vi "OutputSwerveDrive.vi"() -> ()   [LabVIEW 2019]
doc: "This VI runs feedback and feedforward controllers, manages safety interlocks, and sends commands to the swerve drive motors. This VI also controls the commanded driver shifter (low gear or high gear) state."
uses:
  <vilib>/Rock Robotics/WPI/ThirdParty/Phoenix-LabVIEW/Motor Controller/Controls/CTRE_Phoenix_MotorControl_SupplyCurrentLimitConfiguration.ctl
  <vilib>/Rock Robotics/WPI/ThirdParty/Phoenix-LabVIEW/Motor Controller/Controls/CTRE_Phoenix_MotorControl_ControlMode.ctl
  <vilib>/Rock Robotics/WPI/Solenoid/WPI_SolenoidValue.ctl
  5bc46b9e-4d4b-4873-ab3e-533fd441fb60.vi
  eec0778c-44f4-445b-8f09-fbe21d33a92f.vi
  9255c0bb-7061-46f3-9b12-3c6a122af16e.vi
  4c0f1fb3-de9e-41af-b613-55c778746a69.vi
  1feddb54-1091-429e-8d95-9769f01e3028.vi
  9914bed3-0d1c-4b06-b050-22aab9a27a8c.vi
  outputs.vi
  dsdata.vi
  sensors.vi
  refnums.vi
  GRNF_CTREMotor.vi
  <vilib>/Rock Robotics/WPI/ThirdParty/Phoenix-LabVIEW/Motor Controller/Get/CTRE_Phoenix_MotorController_GetSelectedSensorData.vi
  robotprofile.vi
  TAI_Motor.vi
  GRNF_GenericSolenoid.vi
  TAI_Solenoid.vi
  <vilib>/Rock Robotics/WPI/Solenoid/WPI_SolenoidSetEnum.vi
panel:
  in  "Decceleration Limit (/s)":dbl=50.0
  in  "Acceleration Limit (/s)":dbl=2.0
  in  "Force to Low Gear":bool
  in  "Force To High Gear":bool
  in  "Drive Command Override [0,1]":dbl
  in  "Manually Override Drive Calibration":bool
  in  "Time Below Speed (ms)":u32=100
  in  "Time Above Speed (ms)":u32=100
  in  "Switch to Low Gear (rpm)":dbl=740.0
  in  "Switch to High Gear (rpm)":dbl=2000.0
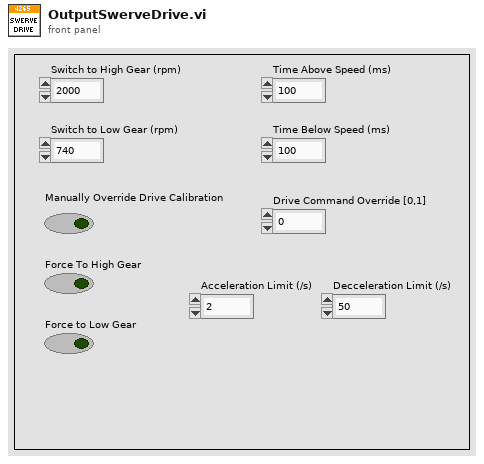
[diagram p1: front panel]
types:
  T1 = enum16{"Driver Control", "Auto Targeting", "Feeder Station"}
  T2 = typedef "CTRE_Phoenix_MotorControl_ControlMode.ctl" = u16
  T3 = typedef "CTRE_Phoenix_MotorControl_SupplyCurrentLimitConfiguration.ctl" = cluster{"Enable?":bool, "Current Limit":dbl, "Threshold Current":dbl, "Threshold Time":dbl}
  T4 = typedef "WPI_MotorControlDeviceRef.ctl" = cluster{"DeviceStatus":errorcluster, "Type":T5, "PWM":cluster{"PWM Channel":T6, "DeadBand":T7}, "CAN":cluster{"Device Number":u8, "SetOutput VI Ref":variant, "GetOutput VI Ref":variant, "Enable VI Ref":variant, "Disable VI Ref":variant, "Data":variant}, "Invert":bool, "DIO PWM":cluster{"PWM \"Enable\" Channel":T6, "DIOChannel":T8, "PWM Rate":dbl}}
  T5 = typedef "WPI_MotorControlType.ctl" = enum16{"PWM", "CAN", "DIO PWM"}
  T6 = typedef "FPGA_DIOPWMChannel.ctl" = enum8{"PWM 0", "PWM 1", "PWM 2", "PWM 3", "PWM 4", "PWM 5", "PWM 6", "PWM 7", "PWM 8", "PWM 9", "PWM MXP 0", "PWM MXP 1", "PWM MXP 2", "PWM MXP 3", "PWM MXP 4", "PWM MXP 5", "PWM MXP 6", "PWM MXP 7", "PWM MXP 8", "PWM MXP 9", "Invalid"}
  T7 = typedef "WPI_PWMDeadband.ctl" = cluster{"Name":string, "maxPositivePwm":i32, "minPositivePwm":i32, "centerPwm":i32, "maxNegativePwm":i32, "minNegativePwm":i32, "angularRange":u16}
  T8 = typedef "FPGA_DIOChannel.ctl" = enum8{"DIO 0", "DIO 1", "DIO 2", "DIO 3", "DIO 4", "DIO 5", "DIO 6", "DIO 7", "DIO 8", "DIO 9", "DIO MXP 0", "DIO MXP 1", "DIO MXP 2", "DIO MXP 3", "DIO MXP 4", "DIO MXP 5", "DIO MXP 6", "DIO MXP 7", "DIO MXP 8", "DIO MXP 9", "DIO MXP 10", "DIO MXP 11", "DIO MXP 12", "DIO MXP 13", "DIO MXP 14", "DIO MXP 15", "SPI Port CS1", "SPI Port CS2", "SPI Port CS3", "SPI Port MISO", "SPI Port MOSI", "Invalid"}
  T9 = enum16{"Low Gear", "High Gear", "Transiting", "Unknown", "Force Low Gear"}
  T10 = typedef "WPI_SolenoidDevRef.ctl" = cluster{"DevStatus":errorcluster, "Pneumatics Control Module":u8, "Forward Solenoid Channel":T11, "Reverse Solenoid Channel":T11}
  T11 = typedef "WPI_SolenoidChannel.ctl" = enum8{"Solenoid 0", "Solenoid 1", "Solenoid 2", "Solenoid 3", "Solenoid 4", "Solenoid 5", "Solenoid 6", "Solenoid 7", "Invalid"}
  T12 = typedef "WPI_SolenoidValue.ctl" = enum16{"Off", "On", "Forward", "Reverse"}
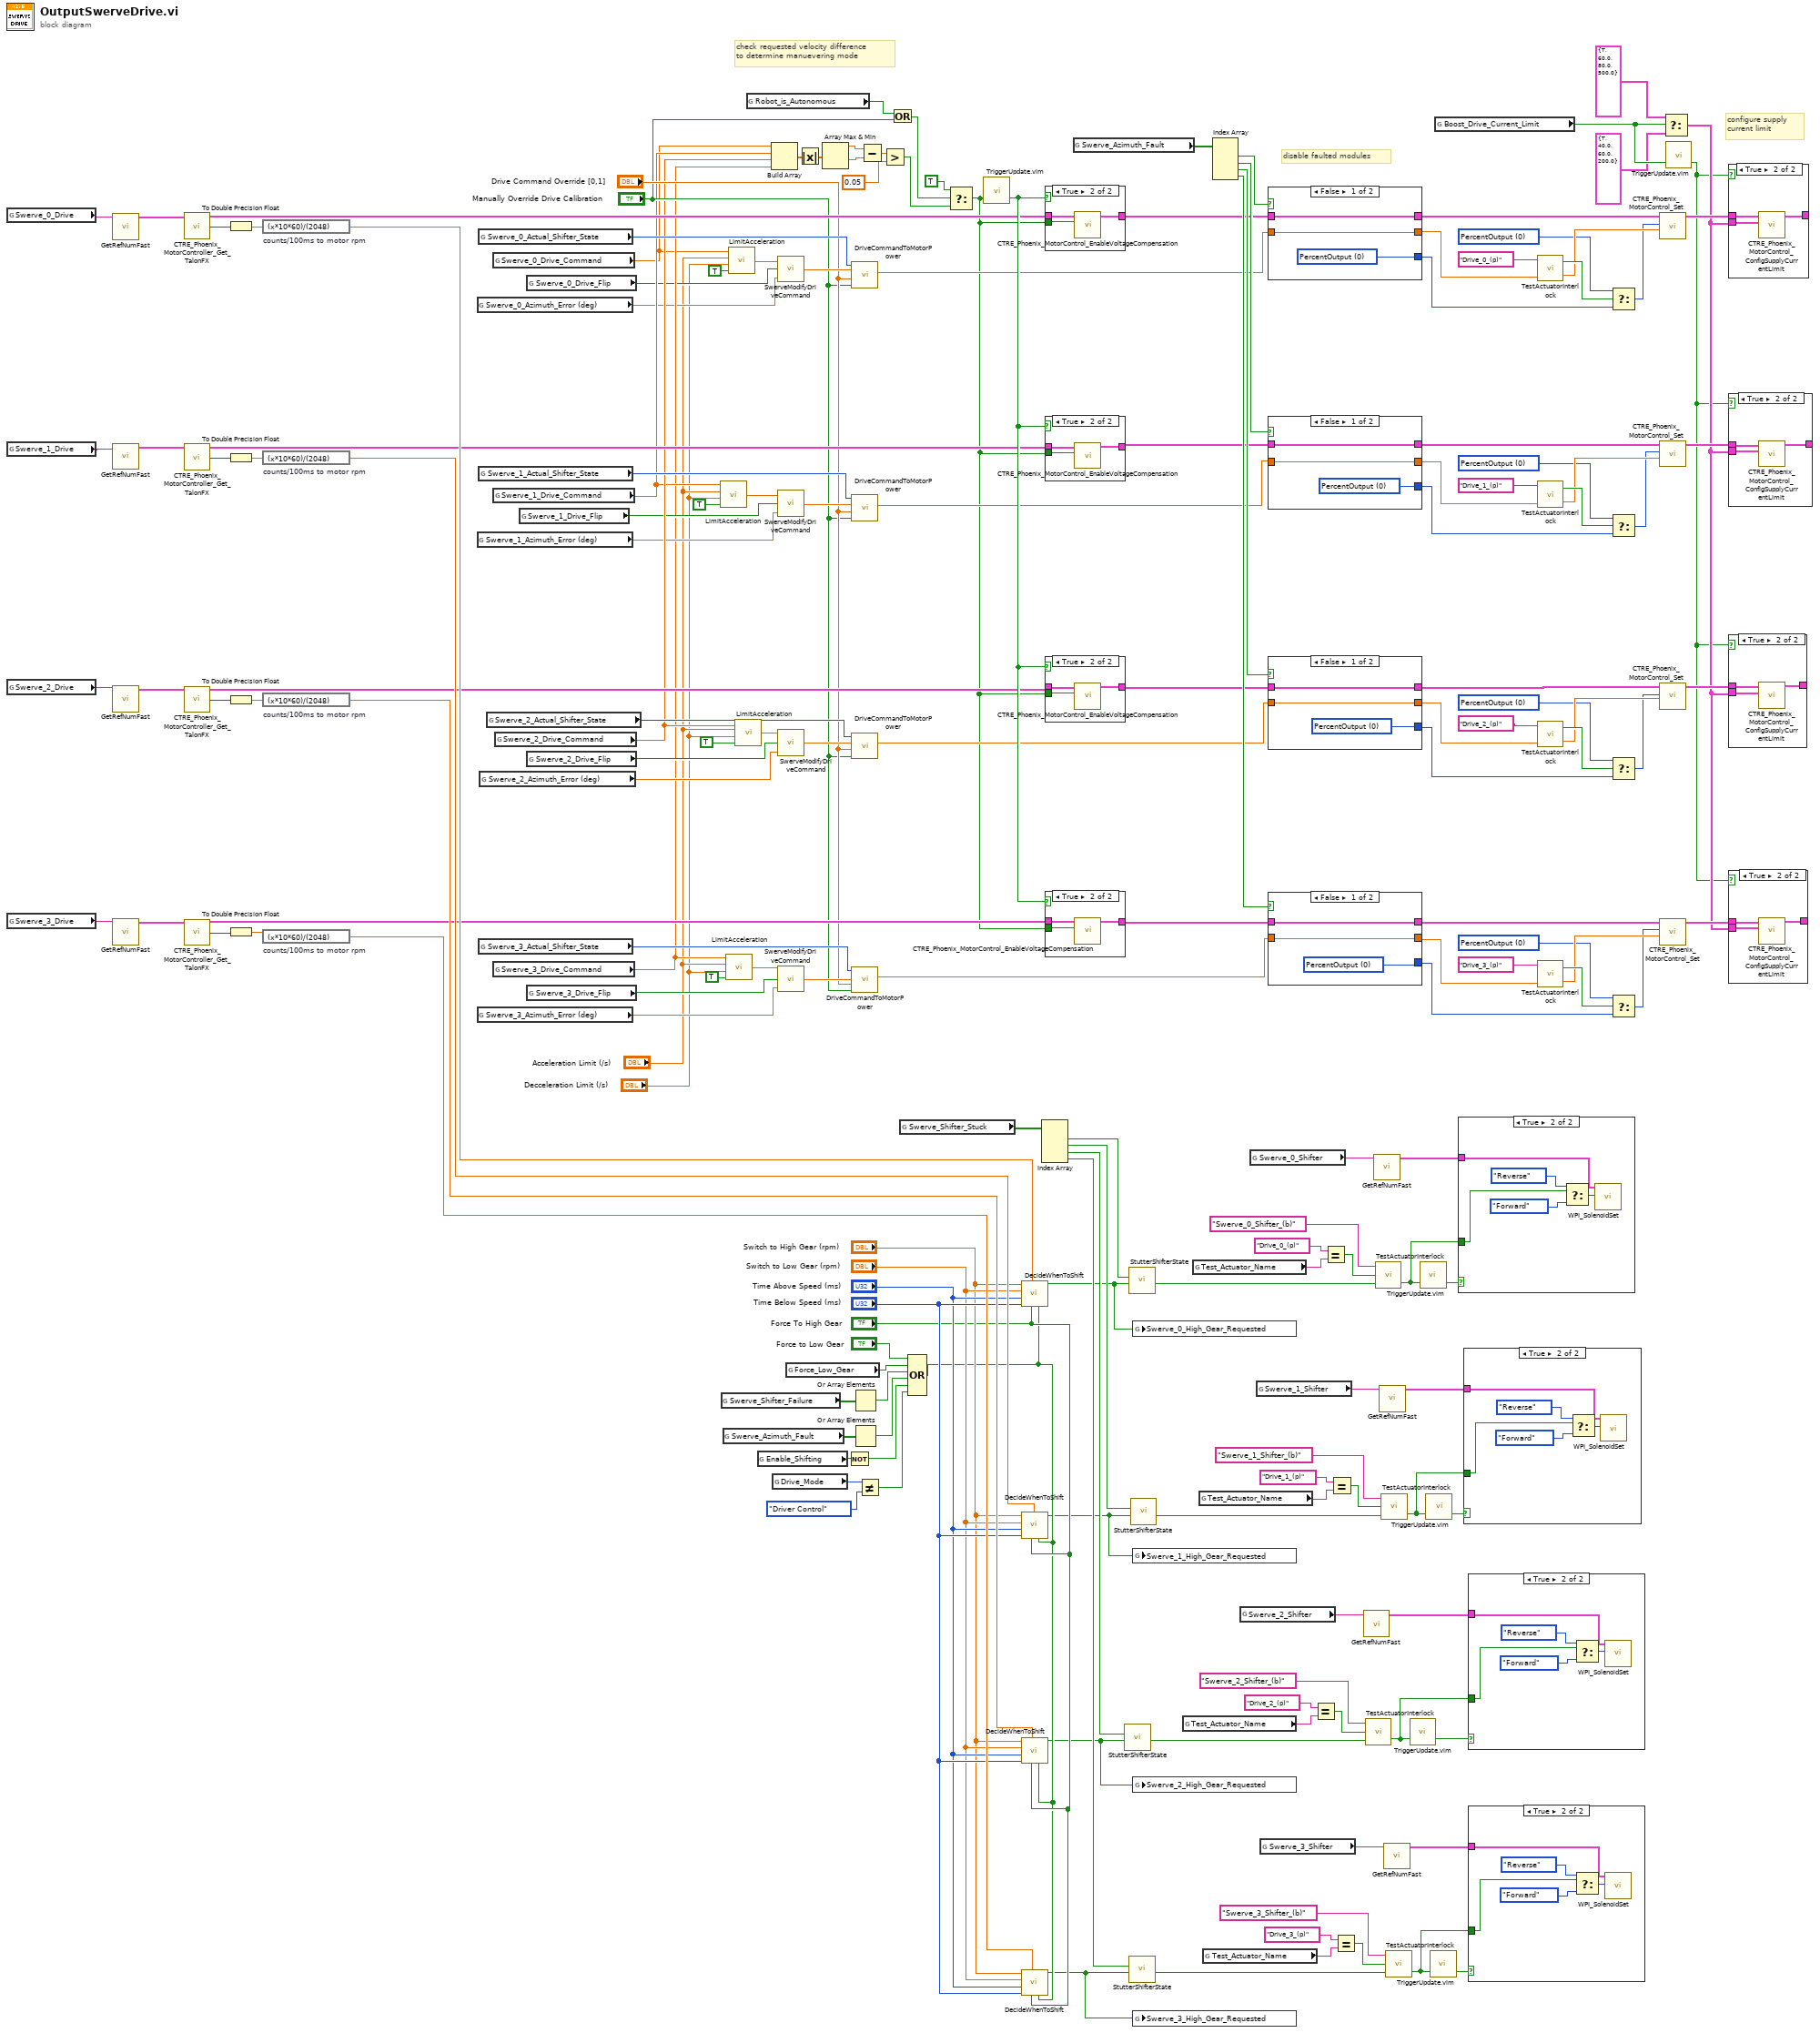
[diagram p0: block diagram]
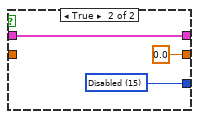
[diagram p14: hidden frame]
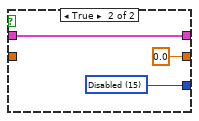
[diagram p15: hidden frame]
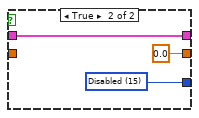
[diagram p16: hidden frame]
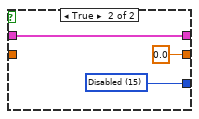
[diagram p17: hidden frame]
diagram:
  w146 = T2 0 items=["PercentOutput"=0, "Position"=1, "Velocity"=2, "Current"=3, "Follower"=5, "MotionProfile"=6, "MotionMagic"=7, "MotionProfileArc"=10, "Disabled"=15] ("Control Mode")
  w155 = T2 0 items=["PercentOutput"=0, "Position"=1, "Velocity"=2, "Current"=3, "Follower"=5, "MotionProfile"=6, "MotionMagic"=7, "MotionProfileArc"=10, "Disabled"=15] ("Control Mode")
  w164 = T2 0 items=["PercentOutput"=0, "Position"=1, "Velocity"=2, "Current"=3, "Follower"=5, "MotionProfile"=6, "MotionMagic"=7, "MotionProfileArc"=10, "Disabled"=15] ("Control Mode")
  w173 = T2 0 items=["PercentOutput"=0, "Position"=1, "Velocity"=2, "Current"=3, "Follower"=5, "MotionProfile"=6, "MotionMagic"=7, "MotionProfileArc"=10, "Disabled"=15] ("Control Mode")
  # "check requested velocity difference\nto determine manuevering mode"
  # "configure supply\ncurrent limit"
  # "disable faulted modules"
  n1 = global read "refnums.vi" "Swerve_0_Drive"() -> (w152:string)
  n2 = global read "refnums.vi" "Swerve_1_Drive"() -> (w161:string)
  n3 = global read "refnums.vi" "Swerve_2_Drive"() -> (w170:string)
  n4 = global read "refnums.vi" "Swerve_3_Drive"() -> (w179:string)
  n5 = call-poly "GetRefNumFast.vi"("RefNum Name"=w152) -> ("Device Reference"=w111:T4)  [unwired: 5 in, 1 out]
  n6 = call-poly "GetRefNumFast.vi"("RefNum Name"=w161) -> ("Device Reference"=w110:T4)  [unwired: 5 in, 1 out]
  n7 = call-poly "GetRefNumFast.vi"("RefNum Name"=w170) -> ("Device Reference"=w109:T4)  [unwired: 5 in, 1 out]
  n8 = call-poly "GetRefNumFast.vi"("RefNum Name"=w179) -> ("Device Reference"=w108:T4)  [unwired: 5 in, 1 out]
  n9 = call-poly <vilib>:"CTRE_Phoenix_MotorController_Get_TalonFX.vi"("PhoenixMotorControlDevRef"=w111) -> ("PhoenixMotorControlDevRef"=w114:T4, "Velocity (Raw Sensor Units per 100 ms)"=w119:i32)  [unwired: 11 in, 2 out]
  n10 = call-poly <vilib>:"CTRE_Phoenix_MotorController_Get_TalonFX.vi"("PhoenixMotorControlDevRef"=w110) -> ("PhoenixMotorControlDevRef"=w112:T4, "Velocity (Raw Sensor Units per 100 ms)"=w118:i32)  [unwired: 11 in, 2 out]
  n11 = call-poly <vilib>:"CTRE_Phoenix_MotorController_Get_TalonFX.vi"("PhoenixMotorControlDevRef"=w109) -> ("PhoenixMotorControlDevRef"=w113:T4, "Velocity (Raw Sensor Units per 100 ms)"=w117:i32)  [unwired: 11 in, 2 out]
  n12 = call-poly <vilib>:"CTRE_Phoenix_MotorController_Get_TalonFX.vi"("PhoenixMotorControlDevRef"=w108) -> ("PhoenixMotorControlDevRef"=w103:T4, "Velocity (Raw Sensor Units per 100 ms)"=w116:i32)  [unwired: 11 in, 2 out]
  n13 = To Double Precision Float(number=w119) -> (double precision float=w126:dbl)
  n14 = To Double Precision Float(number=w118) -> (double precision float=w125:dbl)
  n15 = To Double Precision Float(number=w117) -> (double precision float=w124:dbl)
  n16 = To Double Precision Float(number=w116) -> (double precision float=w123:dbl)
  n17 = expression code="(x*10*60)/(2048)" "counts/100ms to motor rpm"(w126) -> (w120:dbl)
  n18 = expression code="(x*10*60)/(2048)" "counts/100ms to motor rpm"(w125) -> (w121:dbl)
  n19 = expression code="(x*10*60)/(2048)" "counts/100ms to motor rpm"(w124) -> (w122:dbl)
  n20 = expression code="(x*10*60)/(2048)" "counts/100ms to motor rpm"(w123) -> (w134:dbl)
  n21 = global read "outputs.vi" "Swerve_0_Azimuth_Error (deg)"() -> (w70:dbl)
  n22 = global read "outputs.vi" "Swerve_1_Azimuth_Error (deg)"() -> (w76:dbl)
  n23 = global read "outputs.vi" "Swerve_3_Azimuth_Error (deg)"() -> (w115:dbl)
  n24 = global read "sensors.vi" "Swerve_0_Actual_Shifter_State"() -> (w99:T9)
  n25 = global read "sensors.vi" "Swerve_1_Actual_Shifter_State"() -> (w96:T9)
  n26 = global read "sensors.vi" "Swerve_3_Actual_Shifter_State"() -> (w90:T9)
  n27 = global read "outputs.vi" "Swerve_2_Azimuth_Error (deg)"() -> (w81:dbl)
  n28 = global read "sensors.vi" "Swerve_2_Actual_Shifter_State"() -> (w94:T9)
  n29 = global read "outputs.vi" "Swerve_0_Drive_Command"() -> (w67:dbl)
  n30 = global read "outputs.vi" "Swerve_1_Drive_Command"() -> (w75:dbl)
  n31 = global read "outputs.vi" "Swerve_3_Drive_Command"() -> (w72:dbl)
  n32 = global read "outputs.vi" "Swerve_2_Drive_Command"() -> (w84:dbl)
  n33 = global read "outputs.vi" "Swerve_1_Drive_Flip"() -> (w78:bool)
  n34 = global read "outputs.vi" "Swerve_0_Drive_Flip"() -> (w69:bool)
  n35 = global read "outputs.vi" "Swerve_2_Drive_Flip"() -> (w79:bool)
  n36 = global read "outputs.vi" "Swerve_3_Drive_Flip"() -> (w74:bool)
  n37 = call "LimitAcceleration.vi"("Apply Limit"=TRUE, "Decceleration Limit (/s)"="Decceleration Limit (/s)", "Acceleration Limit (/s)"="Acceleration Limit (/s)", "Raw Input"=w75) -> ("Output"=w77:dbl)
  n38 = global read "sensors.vi" "Swerve_Shifter_Failure"() -> (w23:bool[])
  n39 = global read "sensors.vi" "Swerve_Azimuth_Fault"() -> (w21:bool[])
  n40 = call "LimitAcceleration.vi"("Apply Limit"=TRUE, "Decceleration Limit (/s)"="Decceleration Limit (/s)", "Acceleration Limit (/s)"="Acceleration Limit (/s)", "Raw Input"=w72) -> ("Output"=w73:dbl)
  n41 = call "LimitAcceleration.vi"("Apply Limit"=TRUE, "Decceleration Limit (/s)"="Decceleration Limit (/s)", "Acceleration Limit (/s)"="Acceleration Limit (/s)", "Raw Input"=w67) -> ("Output"=w68:dbl)
  n42 = call "LimitAcceleration.vi"("Apply Limit"=TRUE, "Decceleration Limit (/s)"="Decceleration Limit (/s)", "Acceleration Limit (/s)"="Acceleration Limit (/s)", "Raw Input"=w84) -> ("Output"=w82:dbl)
  n43 = global read "dsdata.vi" "Robot_is_Autonomous"() -> (w86:bool)
  n44 = global read "robotprofile.vi" "Enable_Shifting"() -> (w10:bool)
  n45 = Build Array(w67, w75, w84, w72) -> (w133:dbl[])
  n46 = global read "outputs.vi" "Drive_Mode"() -> (w3:T1)
  n47 = call "SwerveModifyDriveCommand.vi"("Azimuth Error (deg)"=w70, "Flip Drive Command"=w69, "Raw Drive Command (ul)"=w68) -> ("Modified Drive Command (ul)"=w100:dbl)
  n48 = call "SwerveModifyDriveCommand.vi"("Azimuth Error (deg)"=w76, "Flip Drive Command"=w78, "Raw Drive Command (ul)"=w77) -> ("Modified Drive Command (ul)"=w97:dbl)
  n49 = call "SwerveModifyDriveCommand.vi"("Azimuth Error (deg)"=w81, "Flip Drive Command"=w79, "Raw Drive Command (ul)"=w82) -> ("Modified Drive Command (ul)"=w93:dbl)
  n50 = call "SwerveModifyDriveCommand.vi"("Azimuth Error (deg)"=w115, "Flip Drive Command"=w74, "Raw Drive Command (ul)"=w73) -> ("Modified Drive Command (ul)"=w91:dbl)
  n51 = global read "outputs.vi" "Force_Low_Gear"() -> (w24:bool)
  n52 = Absolute Value(x=w133) -> (abs(x)=w127:dbl[])
  n53 = Array Max & Min(array=w127) -> (max value=w132:dbl, min value=w131:dbl)  [unwired: 2 out]
  n54 = Not(x=w10) -> (.not. x?=w9:bool)
  n55 = call "DriveCommandToMotorPower.vi"("Drive Command Override"="Manually Override Drive Calibration", "Drive Command Override (ul) [-1,1]"="Drive Command Override [0,1]", "Drive Command (ul) [-1,1]"=w100, "Actual Shifter State"=w99) -> ("Motor Power (ul) [-1,1]"=w98:dbl)  [unwired: 7 in]
  n56 = call "DriveCommandToMotorPower.vi"("Drive Command Override"="Manually Override Drive Calibration", "Drive Command Override (ul) [-1,1]"="Drive Command Override [0,1]", "Drive Command (ul) [-1,1]"=w97, "Actual Shifter State"=w96) -> ("Motor Power (ul) [-1,1]"=w95:dbl)  [unwired: 7 in]
  n57 = call "DriveCommandToMotorPower.vi"("Drive Command Override"="Manually Override Drive Calibration", "Drive Command Override (ul) [-1,1]"="Drive Command Override [0,1]", "Drive Command (ul) [-1,1]"=w93, "Actual Shifter State"=w94) -> ("Motor Power (ul) [-1,1]"=w92:dbl)  [unwired: 7 in]
  n58 = call "DriveCommandToMotorPower.vi"("Drive Command Override"="Manually Override Drive Calibration", "Drive Command Override (ul) [-1,1]"="Drive Command Override [0,1]", "Drive Command (ul) [-1,1]"=w91, "Actual Shifter State"=w90) -> ("Motor Power (ul) [-1,1]"=w89:dbl)  [unwired: 7 in]
  n59 = Or Array Elements(Boolean array=w23) -> (logical OR=w22:bool)
  n60 = Or Array Elements(Boolean array=w21) -> (logical OR=w20:bool)
  n61 = Not Equal?(x=w3, y=T1."Driver Control") -> (x != y?=w1:bool)
  n62 = Subtract(x=w132, y=w131) -> (x-y=w130:dbl)
  n63 = Greater?(x=w130, y=0.05) -> (0:w101:bool)
  n64 = Or(x=w86, y="Manually Override Drive Calibration") -> (x .or. y?=w87:bool)
  n65 = global read "sensors.vi" "Swerve_Shifter_Stuck"() -> (w18:bool[])
  n66 = Compound Arithmetic op=OR("Force to Low Gear", w24, w22, w20, w9, w1) -> (w25:bool)
  n67 = Select(t=TRUE, s=w87, f=w101) -> (s? t:f=w4:bool)
  n68 = call "TriggerUpdate.vim"("Trigger"=w4) -> ("Update"=w128:bool)  [unwired: 2 in]
  n69 = call "DecideWhenToShift.vi"("Force to Low Gear"=w25, "Force To High Gear"="Force To High Gear", "Drive Motor Speed (rpm)"=w120, "Time Below Speed (ms)"="Time Below Speed (ms)", "Time Above Speed (ms)"="Time Above Speed (ms)", "Switch to Low Gear (rpm)"="Switch to Low Gear (rpm)", "Switch to High Gear (rpm)"="Switch to High Gear (rpm)") -> ("Requested Shifter State"=w7:bool)  [unwired: 4 in]
  n70 = call "DecideWhenToShift.vi"("Force to Low Gear"=w25, "Force To High Gear"="Force To High Gear", "Drive Motor Speed (rpm)"=w121, "Time Below Speed (ms)"="Time Below Speed (ms)", "Time Above Speed (ms)"="Time Above Speed (ms)", "Switch to Low Gear (rpm)"="Switch to Low Gear (rpm)", "Switch to High Gear (rpm)"="Switch to High Gear (rpm)") -> ("Requested Shifter State"=w8:bool)  [unwired: 4 in]
  n71 = call "DecideWhenToShift.vi"("Force to Low Gear"=w25, "Force To High Gear"="Force To High Gear", "Drive Motor Speed (rpm)"=w122, "Time Below Speed (ms)"="Time Below Speed (ms)", "Time Above Speed (ms)"="Time Above Speed (ms)", "Switch to Low Gear (rpm)"="Switch to Low Gear (rpm)", "Switch to High Gear (rpm)"="Switch to High Gear (rpm)") -> ("Requested Shifter State"=w6:bool)  [unwired: 4 in]
  n72 = call "DecideWhenToShift.vi"("Force to Low Gear"=w25, "Force To High Gear"="Force To High Gear", "Drive Motor Speed (rpm)"=w134, "Time Below Speed (ms)"="Time Below Speed (ms)", "Time Above Speed (ms)"="Time Above Speed (ms)", "Switch to Low Gear (rpm)"="Switch to Low Gear (rpm)", "Switch to High Gear (rpm)"="Switch to High Gear (rpm)") -> ("Requested Shifter State"=w5:bool)  [unwired: 4 in]
  n73 = Index Array(array=w18) -> (element #1=w16:bool, element #2=w14:bool, element #3=w13:bool, element #4=w11:bool)  [unwired: 4 in]
  n74 = case shown="True" w128 {
    tunnel: w114 -> [w185 w188]
    tunnel: [w185 w187] -> w107
    tunnel: w4 -> [_ w186]
    frame False {
    }
    frame True {
      n75 = call <vilib>:"CTRE_Phoenix_MotorControl_EnableVoltageCompensation.vi"("Enable Voltage Compensation?"=w186, "PhoenixMotorControlDevRef"=w188) -> ("PhoenixMotorControlDevRef"=w187:T4)  [unwired: 8 in, 1 out]
    }
  }
  n76 = case shown="True" w128 {
    tunnel: w112 -> [w189 w192]
    tunnel: [w189 w191] -> w106
    tunnel: w4 -> [_ w190]
    frame False {
    }
    frame True {
      n77 = call <vilib>:"CTRE_Phoenix_MotorControl_EnableVoltageCompensation.vi"("Enable Voltage Compensation?"=w190, "PhoenixMotorControlDevRef"=w192) -> ("PhoenixMotorControlDevRef"=w191:T4)  [unwired: 8 in, 1 out]
    }
  }
  n78 = case shown="True" w128 {
    tunnel: w113 -> [w193 w196]
    tunnel: [w193 w195] -> w105
    tunnel: w4 -> [_ w194]
    frame False {
    }
    frame True {
      n79 = call <vilib>:"CTRE_Phoenix_MotorControl_EnableVoltageCompensation.vi"("Enable Voltage Compensation?"=w194, "PhoenixMotorControlDevRef"=w196) -> ("PhoenixMotorControlDevRef"=w195:T4)  [unwired: 8 in, 1 out]
    }
  }
  n80 = case shown="True" w128 {
    tunnel: [w197 w200] -> w104
    tunnel: w4 -> [_ w199]
    tunnel: w103 -> [w197 w198]
    frame False {
    }
    frame True {
      n81 = call <vilib>:"CTRE_Phoenix_MotorControl_EnableVoltageCompensation.vi"("Enable Voltage Compensation?"=w199, "PhoenixMotorControlDevRef"=w198) -> ("PhoenixMotorControlDevRef"=w200:T4)  [unwired: 8 in, 1 out]
    }
  }
  n82 = global read "sensors.vi" "Swerve_Azimuth_Fault"() -> (w184:bool[])
  n83 = call "StutterShifterState.vi"("Requested Shifter State"=w6, "Request Stutter"=w13) -> ("Stuttered Shifter State"=w19:bool)  [unwired: 9 in]
  n84 = call "StutterShifterState.vi"("Requested Shifter State"=w7, "Request Stutter"=w16) -> ("Stuttered Shifter State"=w17:bool)  [unwired: 9 in]
  n85 = call "StutterShifterState.vi"("Requested Shifter State"=w5, "Request Stutter"=w11) -> ("Stuttered Shifter State"=w12:bool)  [unwired: 9 in]
  n86 = call "StutterShifterState.vi"("Requested Shifter State"=w8, "Request Stutter"=w14) -> ("Stuttered Shifter State"=w15:bool)  [unwired: 9 in]
  n87 = global write "outputs.vi" "Swerve_0_High_Gear_Requested"(w7) -> ()
  n88 = global write "outputs.vi" "Swerve_1_High_Gear_Requested"(w8) -> ()
  n89 = global write "outputs.vi" "Swerve_2_High_Gear_Requested"(w6) -> ()
  n90 = global write "outputs.vi" "Swerve_3_High_Gear_Requested"(w5) -> ()
  n91 = global read "dsdata.vi" "Test_Actuator_Name"() -> (w41:string)
  n92 = global read "dsdata.vi" "Test_Actuator_Name"() -> (w57:string)
  n93 = global read "dsdata.vi" "Test_Actuator_Name"() -> (w49:string)
  n94 = global read "dsdata.vi" "Test_Actuator_Name"() -> (w33:string)
  n95 = Index Array(array=w184) -> (element #1=w143:bool, element #2=w142:bool, element #3=w141:bool, element #4=w183:bool)  [unwired: 4 in]
  n96 = global read "refnums.vi" "Swerve_2_Shifter"() -> (w43:string)
  n97 = global read "refnums.vi" "Swerve_0_Shifter"() -> (w59:string)
  n98 = global read "refnums.vi" "Swerve_1_Shifter"() -> (w51:string)
  n99 = global read "refnums.vi" "Swerve_3_Shifter"() -> (w35:string)
  n100 = case shown="False" w143 {
    tunnel: [w203 w206] -> w151
    tunnel: w107 -> [w203 w206]
    tunnel: [w202 0.0 ("Command")] -> w148
    tunnel: w98 -> [w202 _]
    tunnel: [w201 w204] -> w145
    frame False {
      w201 = T2 0 items=["PercentOutput"=0, "Position"=1, "Velocity"=2, "Current"=3, "Follower"=5, "MotionProfile"=6, "MotionMagic"=7, "MotionProfileArc"=10, "Disabled"=15] ("Control Mode")
    }
    frame True {
      w204 = T2 15 items=["PercentOutput"=0, "Position"=1, "Velocity"=2, "Current"=3, "Follower"=5, "MotionProfile"=6, "MotionMagic"=7, "MotionProfileArc"=10, "Disabled"=15] ("Control Mode")
    }
  }
  n101 = case shown="False" w142 {
    tunnel: [w209 w212] -> w160
    tunnel: w106 -> [w209 w212]
    tunnel: [w208 0.0 ("Command")] -> w157
    tunnel: w95 -> [w208 _]
    tunnel: [w207 w210] -> w154
    frame False {
      w207 = T2 0 items=["PercentOutput"=0, "Position"=1, "Velocity"=2, "Current"=3, "Follower"=5, "MotionProfile"=6, "MotionMagic"=7, "MotionProfileArc"=10, "Disabled"=15] ("Control Mode")
    }
    frame True {
      w210 = T2 15 items=["PercentOutput"=0, "Position"=1, "Velocity"=2, "Current"=3, "Follower"=5, "MotionProfile"=6, "MotionMagic"=7, "MotionProfileArc"=10, "Disabled"=15] ("Control Mode")
    }
  }
  n102 = case shown="False" w141 {
    tunnel: [w215 w218] -> w169
    tunnel: w105 -> [w215 w218]
    tunnel: [w214 0.0 ("Command")] -> w166
    tunnel: w92 -> [w214 _]
    tunnel: [w213 w216] -> w163
    frame False {
      w213 = T2 0 items=["PercentOutput"=0, "Position"=1, "Velocity"=2, "Current"=3, "Follower"=5, "MotionProfile"=6, "MotionMagic"=7, "MotionProfileArc"=10, "Disabled"=15] ("Control Mode")
    }
    frame True {
      w216 = T2 15 items=["PercentOutput"=0, "Position"=1, "Velocity"=2, "Current"=3, "Follower"=5, "MotionProfile"=6, "MotionMagic"=7, "MotionProfileArc"=10, "Disabled"=15] ("Control Mode")
    }
  }
  n103 = case shown="False" w183 {
    tunnel: [w221 w224] -> w178
    tunnel: w104 -> [w221 w224]
    tunnel: [w220 0.0 ("Command")] -> w175
    tunnel: w89 -> [w220 _]
    tunnel: [w219 w222] -> w172
    frame False {
      w219 = T2 0 items=["PercentOutput"=0, "Position"=1, "Velocity"=2, "Current"=3, "Follower"=5, "MotionProfile"=6, "MotionMagic"=7, "MotionProfileArc"=10, "Disabled"=15] ("Control Mode")
    }
    frame True {
      w222 = T2 15 items=["PercentOutput"=0, "Position"=1, "Velocity"=2, "Current"=3, "Follower"=5, "MotionProfile"=6, "MotionMagic"=7, "MotionProfileArc"=10, "Disabled"=15] ("Control Mode")
    }
  }
  n104 = Equal?(x="Drive_2_(p)" ("Actuator_Name"), y=w41) -> (x = y?=w40:bool)
  n105 = Equal?(x="Drive_0_(p)" ("Actuator_Name"), y=w57) -> (x = y?=w56:bool)
  n106 = Equal?(x="Drive_1_(p)" ("Actuator_Name"), y=w49) -> (x = y?=w48:bool)
  n107 = Equal?(x="Drive_3_(p)" ("Actuator_Name"), y=w33) -> (x = y?=w32:bool)
  n108 = call-poly "GetRefNumFast.vi"("RefNum Name"=w43) -> ("Device Reference"=w45:T10)  [unwired: 5 in, 1 out]
  n109 = call-poly "TestActuatorInterlock.vi"("Normal Output"=w19, "Override Actuator Bypass"=w40, "Actuator Name"="Swerve_2_Shifter_(b)" ("Actuator_Name")) -> ("Interlock Output"=w46:bool)  [unwired: 1 out]
  n110 = call-poly "GetRefNumFast.vi"("RefNum Name"=w59) -> ("Device Reference"=w61:T10)  [unwired: 5 in, 1 out]
  n111 = call-poly "TestActuatorInterlock.vi"("Normal Output"=w17, "Override Actuator Bypass"=w56, "Actuator Name"="Swerve_0_Shifter_(b)" ("Actuator_Name")) -> ("Interlock Output"=w62:bool)  [unwired: 1 out]
  n112 = call-poly "GetRefNumFast.vi"("RefNum Name"=w51) -> ("Device Reference"=w53:T10)  [unwired: 5 in, 1 out]
  n113 = call-poly "TestActuatorInterlock.vi"("Normal Output"=w15, "Override Actuator Bypass"=w48, "Actuator Name"="Swerve_1_Shifter_(b)" ("Actuator_Name")) -> ("Interlock Output"=w54:bool)  [unwired: 1 out]
  n114 = call-poly "GetRefNumFast.vi"("RefNum Name"=w35) -> ("Device Reference"=w37:T10)  [unwired: 5 in, 1 out]
  n115 = call-poly "TestActuatorInterlock.vi"("Normal Output"=w12, "Override Actuator Bypass"=w32, "Actuator Name"="Swerve_3_Shifter_(b)" ("Actuator_Name")) -> ("Interlock Output"=w38:bool)  [unwired: 1 out]
  n116 = call "TriggerUpdate.vim"("Trigger"=w46) -> ("Update"=w47:bool)  [unwired: 2 in]
  n117 = call "TriggerUpdate.vim"("Trigger"=w62) -> ("Update"=w63:bool)  [unwired: 2 in]
  n118 = call "TriggerUpdate.vim"("Trigger"=w54) -> ("Update"=w55:bool)  [unwired: 2 in]
  n119 = call "TriggerUpdate.vim"("Trigger"=w38) -> ("Update"=w39:bool)  [unwired: 2 in]
  n120 = global read "outputs.vi" "Boost_Drive_Current_Limit"() -> (w181:bool)
  n121 = case shown="True" w63 {
    tunnel: w61 -> [_ w229]
    tunnel: w62 -> [_ w228]
    frame False {
    }
    frame True {
      n122 = Select(t=WPI_SolenoidValue."Reverse" ("Value"), s=w228, f=WPI_SolenoidValue."Forward" ("Value")) -> (s? t:f=w225:T12)
      n123 = call-poly <vilib>:"WPI_SolenoidSet.vi"("Value"=w225, "SolenoidDevRef"=w229) -> ()  [unwired: 8 in, 2 out]
    }
  }
  n124 = case shown="True" w55 {
    tunnel: w53 -> [_ w234]
    tunnel: w54 -> [_ w233]
    frame False {
    }
    frame True {
      n125 = Select(t=WPI_SolenoidValue."Reverse" ("Value"), s=w233, f=WPI_SolenoidValue."Forward" ("Value")) -> (s? t:f=w230:T12)
      n126 = call-poly <vilib>:"WPI_SolenoidSet.vi"("Value"=w230, "SolenoidDevRef"=w234) -> ()  [unwired: 8 in, 2 out]
    }
  }
  n127 = case shown="True" w47 {
    tunnel: w45 -> [_ w239]
    tunnel: w46 -> [_ w238]
    frame False {
    }
    frame True {
      n128 = Select(t=WPI_SolenoidValue."Reverse" ("Value"), s=w238, f=WPI_SolenoidValue."Forward" ("Value")) -> (s? t:f=w235:T12)
      n129 = call-poly <vilib>:"WPI_SolenoidSet.vi"("Value"=w235, "SolenoidDevRef"=w239) -> ()  [unwired: 8 in, 2 out]
    }
  }
  n130 = case shown="True" w39 {
    tunnel: w37 -> [_ w244]
    tunnel: w38 -> [_ w243]
    frame False {
    }
    frame True {
      n131 = Select(t=WPI_SolenoidValue."Reverse" ("Value"), s=w243, f=WPI_SolenoidValue."Forward" ("Value")) -> (s? t:f=w240:T12)
      n132 = call-poly <vilib>:"WPI_SolenoidSet.vi"("Value"=w240, "SolenoidDevRef"=w244) -> ()  [unwired: 8 in, 2 out]
    }
  }
  n133 = call-poly "TestActuatorInterlock.vi"("Normal Output"=w148, "Actuator Name"="Drive_0_(p)" ("Actuator_Name")) -> ("Interlock Output"=w147:dbl, "Testing This Actuator"=w150:bool)  [unwired: 1 in]
  n134 = call-poly "TestActuatorInterlock.vi"("Normal Output"=w157, "Actuator Name"="Drive_1_(p)" ("Actuator_Name")) -> ("Interlock Output"=w156:dbl, "Testing This Actuator"=w159:bool)  [unwired: 1 in]
  n135 = call-poly "TestActuatorInterlock.vi"("Normal Output"=w166, "Actuator Name"="Drive_2_(p)" ("Actuator_Name")) -> ("Interlock Output"=w165:dbl, "Testing This Actuator"=w168:bool)  [unwired: 1 in]
  n136 = call-poly "TestActuatorInterlock.vi"("Normal Output"=w175, "Actuator Name"="Drive_3_(p)" ("Actuator_Name")) -> ("Interlock Output"=w174:dbl, "Testing This Actuator"=w177:bool)  [unwired: 1 in]
  n137 = Select(t=w146, s=w150, f=w145) -> (s? t:f=w144:T2)
  n138 = Select(t=w155, s=w159, f=w154) -> (s? t:f=w153:T2)
  n139 = Select(t=w164, s=w168, f=w163) -> (s? t:f=w162:T2)
  n140 = Select(t=w173, s=w177, f=w172) -> (s? t:f=w171:T2)
  n141 = call <vilib>:"CTRE_Phoenix_MotorControl_Set.vi"("Output"=w147, "Control Mode"=w144, "PhoenixMotorControlDevRef"=w151) -> ("PhoenixMotorControlDevRef"=w140:T4)  [unwired: 7 in, 1 out]
  n142 = call <vilib>:"CTRE_Phoenix_MotorControl_Set.vi"("Output"=w156, "Control Mode"=w153, "PhoenixMotorControlDevRef"=w160) -> ("PhoenixMotorControlDevRef"=w139:T4)  [unwired: 7 in, 1 out]
  n143 = call <vilib>:"CTRE_Phoenix_MotorControl_Set.vi"("Output"=w165, "Control Mode"=w162, "PhoenixMotorControlDevRef"=w169) -> ("PhoenixMotorControlDevRef"=w138:T4)  [unwired: 7 in, 1 out]
  n144 = call <vilib>:"CTRE_Phoenix_MotorControl_Set.vi"("Output"=w174, "Control Mode"=w171, "PhoenixMotorControlDevRef"=w178) -> ("PhoenixMotorControlDevRef"=w137:T4)  [unwired: 7 in, 1 out]
  n145 = Select(t=T3 {"Enable?"=TRUE, "Current Limit"=60.0, "Threshold Current"=80.0, "Threshold Time"=500.0} ("Supply Current Limit Configuration"), s=w181, f=T3 {"Enable?"=TRUE, "Current Limit"=40.0, "Threshold Current"=60.0, "Threshold Time"=200.0} ("Supply Current Limit Configuration")) -> (s? t:f=w136:T3)
  n146 = call "TriggerUpdate.vim"("Trigger"=w181) -> ("Update"=w135:bool)  [unwired: 2 in]
  n147 = case shown="True" w135 {
    tunnel: w140 -> [w245 w248]
    tunnel: [w245 w247] -> _
    tunnel: w136 -> [_ w246]
    frame False {
    }
    frame True {
      n148 = call <vilib>:"CTRE_Phoenix_MotorControl_ConfigSupplyCurrentLimit.vi"("Supply Current Limit Configuration"=w246, "PhoenixMotorControlDevRef"=w248) -> ("PhoenixMotorControlDevRef"=w247:T4)  [unwired: 8 in, 1 out]
    }
  }
  n149 = case shown="True" w135 {
    tunnel: w139 -> [w249 w252]
    tunnel: [w249 w251] -> _
    tunnel: w136 -> [_ w250]
    frame False {
    }
    frame True {
      n150 = call <vilib>:"CTRE_Phoenix_MotorControl_ConfigSupplyCurrentLimit.vi"("Supply Current Limit Configuration"=w250, "PhoenixMotorControlDevRef"=w252) -> ("PhoenixMotorControlDevRef"=w251:T4)  [unwired: 8 in, 1 out]
    }
  }
  n151 = case shown="True" w135 {
    tunnel: w138 -> [w253 w256]
    tunnel: [w253 w255] -> _
    tunnel: w136 -> [_ w254]
    frame False {
    }
    frame True {
      n152 = call <vilib>:"CTRE_Phoenix_MotorControl_ConfigSupplyCurrentLimit.vi"("Supply Current Limit Configuration"=w254, "PhoenixMotorControlDevRef"=w256) -> ("PhoenixMotorControlDevRef"=w255:T4)  [unwired: 8 in, 1 out]
    }
  }
  n153 = case shown="True" w135 {
    tunnel: w137 -> [w257 w260]
    tunnel: [w257 w259] -> _
    tunnel: w136 -> [_ w258]
    frame False {
    }
    frame True {
      n154 = call <vilib>:"CTRE_Phoenix_MotorControl_ConfigSupplyCurrentLimit.vi"("Supply Current Limit Configuration"=w258, "PhoenixMotorControlDevRef"=w260) -> ("PhoenixMotorControlDevRef"=w259:T4)  [unwired: 8 in, 1 out]
    }
  }
